vi "Set Channel.vi"(8 "error in (no error)":errorcluster, 10 "Channel":T1 items=["Channel 0", "Channel 1", "Channel 2", "Channel 3", "Channel 4", "Channel 5", "Channel 6", "Channel 7", "Channel 8", "Channel 9", "Channel 10", "Channel 11", "Channel 12", "Channel 13", "Channel 14", "Channel 15"], 11 "Potentiostat Galvanostat in":refnum<class "Potentiostat Galvanostat.lvclass">) -> (0 "error out":errorcluster, 3 "Potentiostat Galvanostat out":refnum<class "Potentiostat Galvanostat.lvclass">)   [LabVIEW 2018, in "Potentiostat Galvanostat.lvclass"]
uses:
  Potentiostat Galvanostat.lvclass
  Controls/Channel.ctl
  Potentiostat Galvanostat.lvclass/Potentiostat Galvanostat.ctl
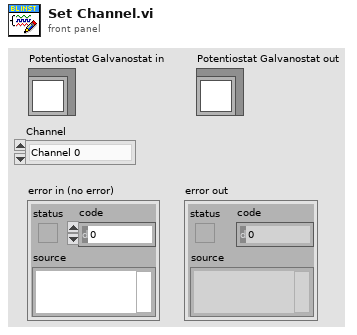
[diagram p1: front panel]
types:
  T1 = typedef "Potentiostat Galvanostat.lvclass/Channel.ctl" = u8
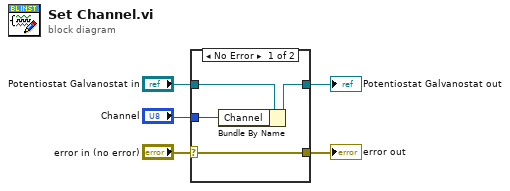
[diagram p0: block diagram]
diagram:
  n1 = case shown="No Error" "error in (no error)" {
    selector: "error in (no error)" -> [w9 w10]
    tunnel: [w9 w10] -> w4
    tunnel: [w7 w11] -> w2
    tunnel: "Potentiostat Galvanostat in" -> [w8 w11]
    tunnel: "Channel" -> [w6 _]
    frame No Error {
      n2 = Bundle By Name(cluster=w8, "Channel"=w6) -> (w7:refnum<class "Potentiostat Galvanostat.lvclass">)
    }
    frame Error {
    }
  }
  "error out" <- w4
  "Potentiostat Galvanostat out" <- w2
